vi "Public Send Launch Nested Actor Msg.vi"(7 "Message Priority (Normal)":T1=enum."Normal", 8 "error in":errorcluster, 9 "Auto-stop? (T)":bool=TRUE, 10 "Nested Actor":refnum<class "Actor.lvclass">, 11 "Self Enqueuer in":refnum<class "Message Enqueuer.lvclass">) -> (0 "error out":errorcluster, 3 "Self Enqueuer out":refnum<class "Message Enqueuer.lvclass">)   [LabVIEW 2017, in "ActorNotifiesWhenStopped.lvclass"]
uses:
  ActorNotifiesWhenStopped.lvclass
  <vilib>/ActorFramework/Message Enqueuer/Message Priority.ctl
  <vilib>/ActorFramework/Actor/Actor.lvclass
  <vilib>/ActorFramework/Message Enqueuer/Message Enqueuer.lvclass
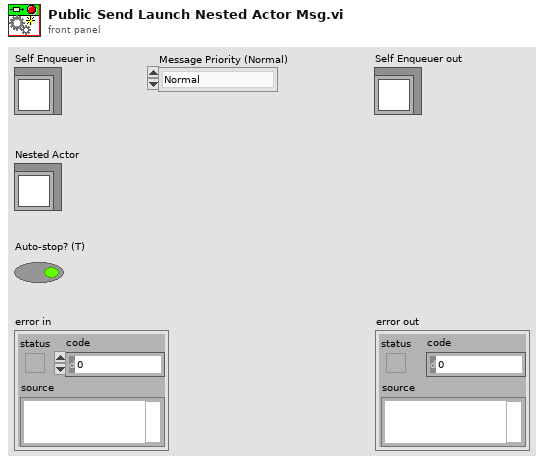
[diagram p1: front panel]
types:
  T1 = typedef "Actor Framework.lvlib/Message Enqueuer.lvclass/Message Priority.ctl" = enum16{"Low", "Normal", "High"}
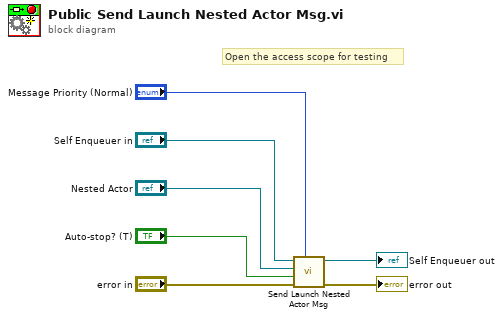
[diagram p0: block diagram]
diagram:
  # "Open the access scope for testing"
  n1 = call <vilib>:"Send Launch Nested Actor Msg.vi"("Message Priority (Normal)"="Message Priority (Normal)", "error in"="error in", "Auto-stop? (T)"="Auto-stop? (T)", "Nested Actor"="Nested Actor", "Self Enqueuer in"="Self Enqueuer in") -> ("error out"=→"error out":errorcluster, "Self Enqueuer out"=→"Self Enqueuer out":refnum<class "Message Enqueuer.lvclass">)  [unwired: 5 in]
